vi "Encoders TestCode.vi"(1 "Step Text":string="String", 2 "Step Text":string="String") -> (8 "Encoders Output":string)   [LabVIEW 2014]
panel:
  in  "Progress Bar":string="Numeric"
  out "Distance Encoder 2":dbl
  out "Distance Encoder 1":dbl
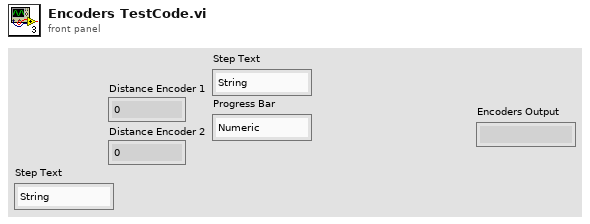
[diagram p1: front panel]
types:
  T1 = typedef "WPI_EncoderDevRef.ctl" = cluster{"DevStatus":errorcluster, "EncoderIndex":T2, "CounterIndex":T3, "DistancePerCount":dbl, "Decoding Type":T4}
  T2 = typedef "FPGA_EncoderIdx.ctl" = enum8{"Enc 0", "Enc 1", "Enc 2", "Enc 3", "Enc 4", "Enc 5", "Enc 6", "Enc 7", "Invalid"}
  T3 = typedef "FPGA_CounterCtrSystemIndex.ctl" = enum8{"Ctr 0", "Ctr 1", "Ctr 2", "Ctr 3", "Ctr 4", "Ctr 5", "Ctr 6", "Ctr 7", "Invalid"}
  T4 = typedef "WPI_EncoderType.ctl" = enum16{"1x", "2x", "4x"}
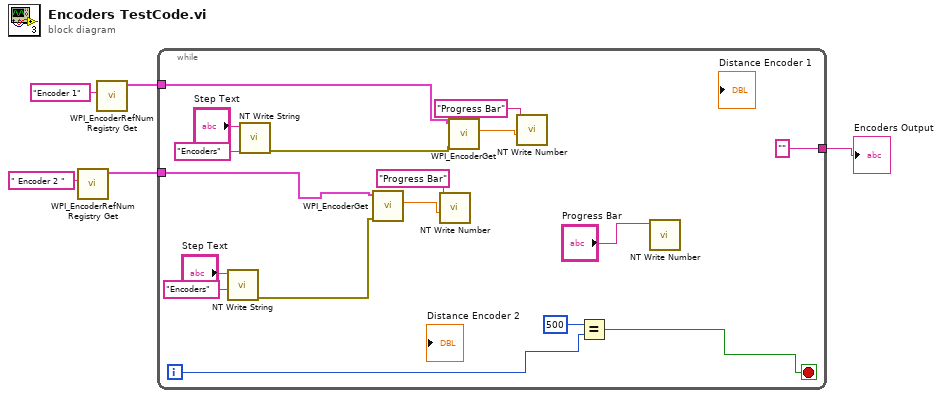
[diagram p0: block diagram]
diagram:
  n1 = call <vilib>:"WPI_EncoderRefNum Registry Get.vi"("refnum name"=" Encoder 2 ") -> ("EncoderDevRef"=w4:T1)  [unwired: 9 in, 1 out]
  n2 = call <vilib>:"WPI_EncoderRefNum Registry Get.vi"("refnum name"="Encoder 1") -> ("EncoderDevRef"=w2:T1)  [unwired: 9 in, 1 out]
  n3 = while {
    tunnel: w4 -> [w11]
    tunnel: w2 -> [w10]
    tunnel: ["" ("Encoders")] -> w1
    i -> [w8]
    stop <- w6 stop-if-true
    n4 = call <vilib>:"NT Write String.vi"("String"="Encoders", "Name"="Step Text") -> ("error out"=w22:errorcluster)  [unwired: 9 in]
    n5 = call <vilib>:"NT Write String.vi"("String"="Encoders", "Name"="Step Text") -> ("error out"=w18:errorcluster)  [unwired: 9 in]
    n6 = call <vilib>:"WPI_EncoderGet.vi"("error in (no error)"=w22, "EncoderDevRef"=w11) -> ("Distance"=w15:dbl)  [unwired: 4 in, 5 out]
    n7 = call <vilib>:"NT Write Number.vi"("Numeric"=w15, "Name"="Progress Bar") -> ()  [unwired: 9 in, 1 out]
    n8 = call <vilib>:"WPI_EncoderGet.vi"("error in (no error)"=w18, "EncoderDevRef"=w10) -> ("Distance"=w13:dbl)  [unwired: 4 in, 5 out]
    n9 = call <vilib>:"NT Write Number.vi"("Numeric"=w13, "Name"="Progress Bar") -> ()  [unwired: 9 in, 1 out]
    n10 = Equal?(x=500, y=w8) -> (x = y?=w6:bool)
    n11 = call <vilib>:"NT Write Number.vi"("Name"="Progress Bar") -> ()  [unwired: 10 in, 1 out]
  }
  "Encoders Output" <- w1
